vi "bulk_read.vi"() -> ()   [LabVIEW 2016]
uses:
  dxl_x86_c.lvlib/dxl_x86_c.lvlib
panel:
  out "dynamixel_comm_result":string
  out "dynamixel_error":string
  in  "LEN_MX_\nMOVING":u16=1
  in  "ADDR_MX_\nMOVING":u16=46
  out "value : MX (LED)\nis moving 2":bool
  out "group_num":i32
  in  "LEN_MX_\nPRESENT_POSITION":u16=2
  in  "dynamixe2_id":u8=2
  in  "device_name":string="COM1"
  in  "ADDR_MX_\nPRESENT_POSITION":u16=36
  in  "ADDR_MX_\nGOAL_POSITION":u16=30
  in  "ADDR_MX_\nTORQUE_ENABLE":u16=24
  out "protocol_version":dbl=1.0
  out "value : MX (knob)\npresent position 1":u32(knob)
  in  "terminate":bool
  out "port_num":i32
  in  "value : MX (dial)\ngoal position":u16(knob)
  in  "dynamixel1_id":u8=1
  in  "baud_rate":i32=57600
  # "/*******************************************************************************\n* Copyright (c) 2016, ROBOTIS CO., LTD.\n* All rights reserved.\n*\n* Redistribution and use in source and binary forms, with or without\n* modification, are permitted provided that the following conditions are met:\n*\n* * Redistributions of source code must retain the above copyright notice, this\n*   list of conditions and the following disclaimer.\n*\n* * Redistributions in binary form must reproduce the above copyright notice,\n*   this list of conditions and the following disclaimer in the documentation\n*   and/or other materials provided with the distribution.\n*\n* * Neither the name of ROBOTIS nor the names of its\n*   contributors may be used to endorse or promote products derived from\n*   this software without specific prior written permission.\n*\n* THIS SOFTWARE IS PROVIDED BY THE COPYRIGHT HOLDERS AND CONTRIBUTORS \"AS IS\"\n* AND ANY EXPRESS OR IMPLIED WARRANTIES, INCLUDING, BUT NOT LIMITED TO, THE\n* IMPLIED WARRANTIES OF MERCHANTABILITY AND FITNESS FOR A PARTICULAR PURPOSE ARE\n* DISCLAIMED. IN NO EVENT SHALL THE COPYRIGHT HOLDER OR CONTRIBUTORS BE LIABLE\n* FOR ANY DIRECT, INDIRECT, INCIDENTAL, SPECIAL, EXEMPLARY, OR CONSEQUENTIAL\n* DAMAGES (INCLUDING, BUT NOT LIMITED TO, PROCUREMENT OF SUBSTITUTE GOODS OR\n* SERVICES; LOSS OF USE, DATA, OR PROFITS; OR BUSINESS INTERRUPTION) HOWEVER\n* CAUSED AND ON ANY THEORY OF LIABILITY, WHETHER IN CONTRACT, STRICT LIABILITY,\n* OR TORT (INCLUDING NEGLIGENCE OR OTHERWISE) ARISING IN ANY WAY OUT OF THE USE\n* OF THIS SOFTWARE, EVEN IF ADVISED OF THE POSSIBILITY OF SUCH DAMAGE.\n*******************************************************************************/\n\n/* Author: Ryu Woon Jung (Leon) */"
  # "Available Dynamixel model on this example : All models using Protocol 1.0\nThis example is designed for using two Dynamixel MX-28s, and an USB2DYNAMIXEL.\nTo use another Dynamixel model, such as X series, see their details in E-Manual(support.robotis.com) \n   and edit \"numeric control\"s seen left with \"Edit Text\" tool.\nBe sure that Dynamixel MX properties are already set as %% ID : 1 / Baudnum : 34 (Baudrate : 57600)\n\n1. Run example by click above \"Run\" button (below \"Edit\" menu).\n2. Drag \"dial\" then you may see the Dynamixel and \"knob\"s rotating\n3. To finish the example, press \"terminate\" button."
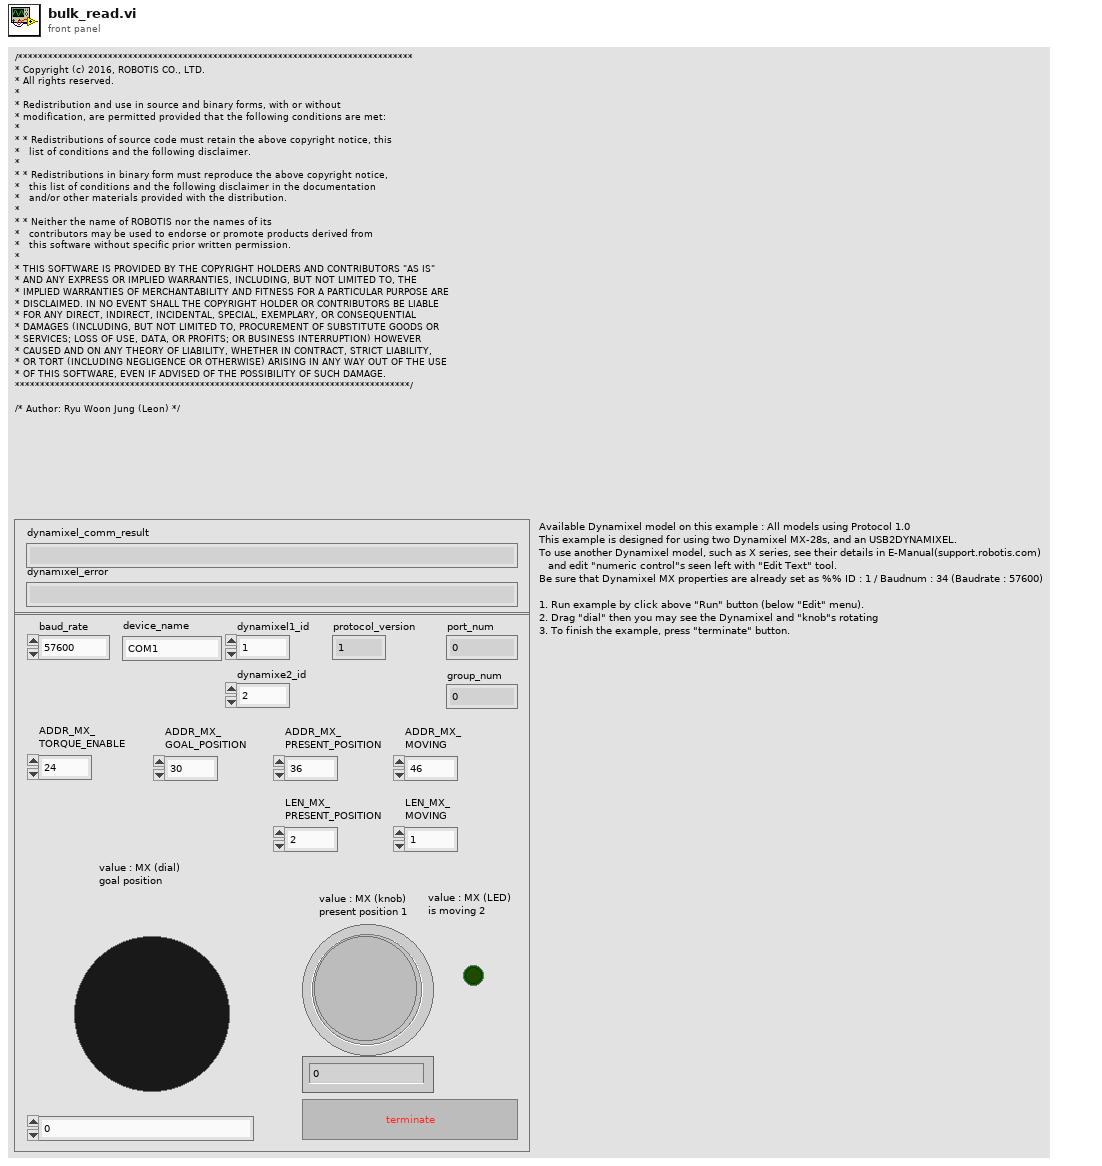
[diagram p1: front panel]
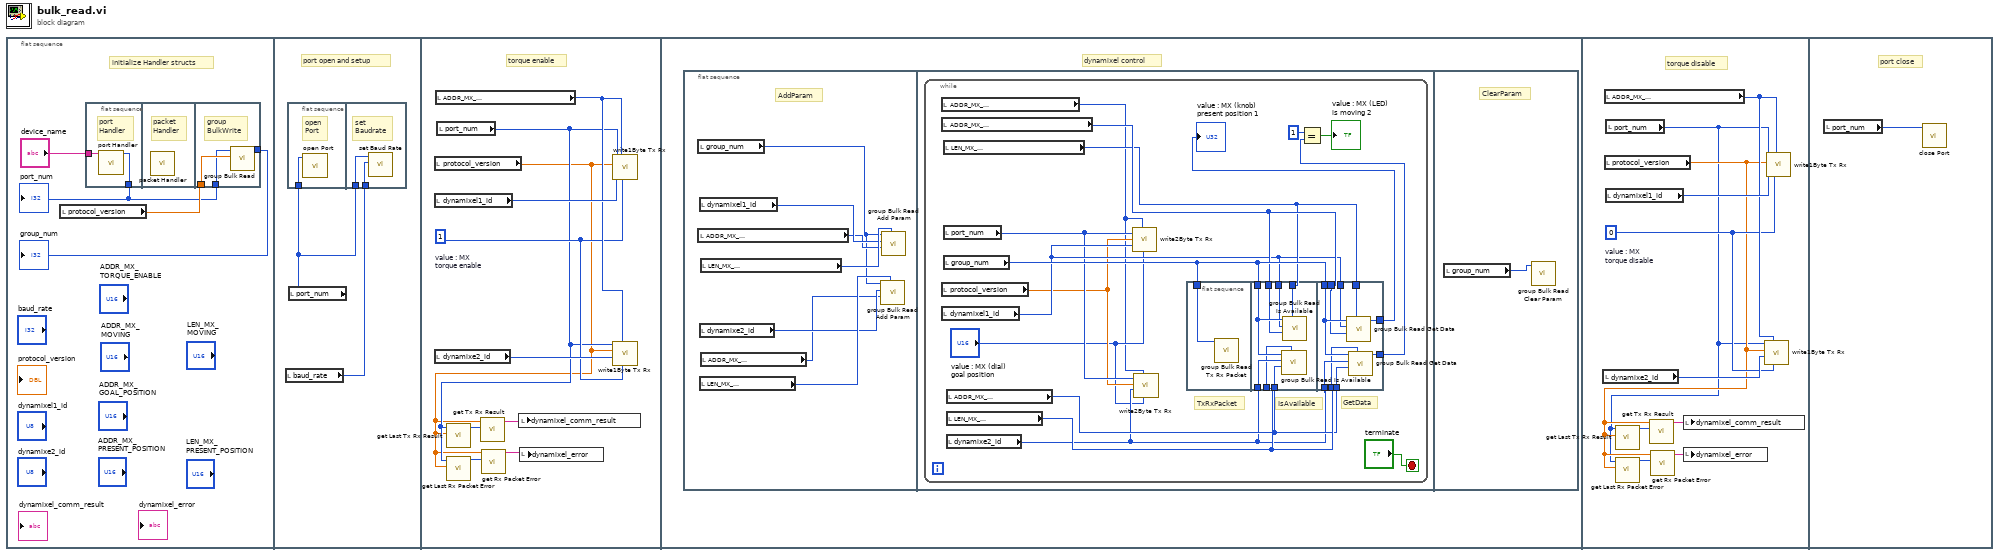
[diagram p0: block diagram]
diagram:
  n1 = flat-sequence {
    frame #0 {
      # "initialize Handler structs"
      n2 = local read "protocol_version"() -> (w3:dbl)
      n3 = flat-sequence {
        tunnel: "device_name" -> [w6]
        tunnel: [w5] -> w2
        tunnel: w3 -> [w9]
        tunnel: w2 -> [w8]
        tunnel: [w7] -> w1
        frame #0 {
          # "port\nHandler"
          n4 = call "port Handler.vi"("port_name"=w6) -> ("function return"=w5:i32)  [unwired: 10 in]
        }
        frame #1 {
          # "packet\nHandler"
          n5 = call "packet Handler.vi"() -> ()  [unwired: 12 in]
        }
        frame #2 {
          # "group\nBulkWrite"
          n6 = call "group Bulk Read.vi"("protocol_version"=w9, "port_num"=w8) -> ("function return"=w7:i32)  [unwired: 9 in]
        }
      }
      "port_num" <- w2
      "group_num" <- w1
    }
    frame #1 {
      # "port open and setup"
      n7 = local read "baud_rate"() -> (w10:i32)
      n8 = flat-sequence {
        tunnel: w11 -> [w12]
        tunnel: w11 -> [w14]
        tunnel: w10 -> [w13]
        frame #0 {
          # "open\nPort"
          n9 = call "open Port.vi"("port_num"=w12) -> ()  [unwired: 10 in, 1 out]
        }
        frame #1 {
          # "set\nBaudrate"
          n10 = call "set Baud Rate.vi"("baudrate"=w13, "port_num"=w14) -> ()  [unwired: 9 in, 1 out]
        }
      }
      n11 = local read "port_num"() -> (w11:i32)
    }
    frame #2 {
      w21 = 1  # value : MX torque enable
      # "torque enable"
      n12 = local read "protocol_version"() -> (w15:dbl)
      n13 = local read "dynamixel1_id"() -> (w24:u8)
      n14 = local read "dynamixe2_id"() -> (w22:u8)
      n15 = local read "ADDR_MX_\nTORQUE_ENABLE"() -> (w23:u16)
      n16 = local read "port_num"() -> (w16:i32)
      n17 = call "get Last Tx Rx Result.vi"("protocol_version"=w15, "port_num"=w16) -> ("function return"=w17:i32)  [unwired: 9 in]
      n18 = call "get Last Rx Packet Error.vi"("protocol_version"=w15, "port_num"=w16) -> ("function return"=w18:u8)  [unwired: 9 in]
      n19 = call "get Tx Rx Result.vi"("result"=w17, "protocol_version"=w15) -> ("function return"=w19:string)  [unwired: 9 in]
      n20 = call "get Rx Packet Error.vi"("error"=w18, "protocol_version"=w15) -> ("function return"=w20:string)  [unwired: 9 in]
      n21 = local write "dynamixel_comm_result"(w19) -> ()
      n22 = local write "dynamixel_error"(w20) -> ()
      n23 = call "write1Byte Tx Rx.vi"("data"=w21, "address"=w23, "id"=w24, "protocol_version"=w15, "port_num"=w16) -> ()  [unwired: 7 in]
      n24 = call "write1Byte Tx Rx.vi"("data"=w21, "address"=w23, "id"=w22, "protocol_version"=w15, "port_num"=w16) -> ()  [unwired: 7 in]
    }
    frame #3 {
      # "dynamixel control"
      n25 = flat-sequence {
        frame #0 {
          # "AddParam"
          n26 = local read "group_num"() -> (w27:i32)
          n27 = local read "ADDR_MX_\nPRESENT_POSITION"() -> (w29:u16)
          n28 = local read "dynamixel1_id"() -> (w30:u8)
          n29 = local read "dynamixe2_id"() -> (w26:u8)
          n30 = local read "LEN_MX_\nMOVING"() -> (w28:u16)
          n31 = local read "LEN_MX_\nPRESENT_POSITION"() -> (w31:u16)
          n32 = local read "ADDR_MX_\nMOVING"() -> (w25:u16)
          n33 = call "group Bulk Read Add Param.vi"("data_length"=w28, "start_address"=w25, "id"=w26, "group_num"=w27) -> ()  [unwired: 7 in, 1 out]
          n34 = call "group Bulk Read Add Param.vi"("data_length"=w31, "start_address"=w29, "id"=w30, "group_num"=w27) -> ()  [unwired: 7 in, 1 out]
        }
        frame #1 {
          n35 = while {
            stop <- "terminate" stop-if-true
            # "TxRxPacket"
            # "IsAvailable"
            # "GetData"
            n36 = local read "ADDR_MX_\nGOAL_POSITION"() -> (w32:u16)
            n37 = local read "ADDR_MX_\nPRESENT_POSITION"() -> (w45:u16)
            n38 = local read "protocol_version"() -> (w35:dbl)
            n39 = local read "dynamixel1_id"() -> (w37:u8)
            n40 = local read "LEN_MX_\nPRESENT_POSITION"() -> (w38:u16)
            n41 = local read "port_num"() -> (w36:i32)
            n42 = local read "group_num"() -> (w46:i32)
            n43 = local read "ADDR_MX_\nMOVING"() -> (w39:u16)
            n44 = local read "LEN_MX_\nMOVING"() -> (w44:u16)
            n45 = local read "dynamixe2_id"() -> (w34:u8)
            n46 = call "write2Byte Tx Rx.vi"("data"="value : MX (dial)\ngoal position", "address"=w32, "id"=w37, "protocol_version"=w35, "port_num"=w36) -> ()  [unwired: 7 in]
            n47 = call "write2Byte Tx Rx.vi"("data"="value : MX (dial)\ngoal position", "address"=w32, "id"=w34, "protocol_version"=w35, "port_num"=w36) -> ()  [unwired: 7 in]
            n48 = flat-sequence {
              tunnel: w46 -> [w48]
              tunnel: w46 -> [w55]
              tunnel: w34 -> [w54]
              tunnel: w45 -> [w53]
              tunnel: w44 -> [w52]
              tunnel: w39 -> [w51]
              tunnel: w38 -> [w50]
              tunnel: w37 -> [w49]
              tunnel: w46 -> [w64]
              tunnel: w34 -> [w63]
              tunnel: w45 -> [w62]
              tunnel: w44 -> [w59]
              tunnel: [w61] -> w41
              tunnel: [w60] -> w40
              tunnel: w39 -> [w58]
              tunnel: w38 -> [w57]
              tunnel: w37 -> [w56]
              frame #0 {
                n49 = call "group Bulk Read Tx Rx Packet.vi"("group_num"=w48) -> ()  [unwired: 11 in]
              }
              frame #1 {
                n50 = call "group Bulk Read Is Available.vi"("data_length"=w52, "address"=w51, "id"=w54, "group_num"=w55) -> ()  [unwired: 7 in, 1 out]
                n51 = call "group Bulk Read Is Available.vi"("data_length"=w50, "address"=w53, "id"=w49, "group_num"=w55) -> ()  [unwired: 7 in, 1 out]
              }
              frame #2 {
                n52 = call "group Bulk Read Get Data.vi"("data_length"=w57, "address"=w62, "id"=w56, "group_num"=w64) -> ("function return"=w60:u32)  [unwired: 7 in]
                n53 = call "group Bulk Read Get Data.vi"("data_length"=w59, "address"=w58, "id"=w63, "group_num"=w64) -> ("function return"=w61:u32)  [unwired: 7 in]
              }
            }
            n54 = Equal?(x=1, y=w41) -> (x = y?=→"value : MX (LED)\nis moving 2":bool)
            "value : MX (knob)\npresent position 1" <- w40
          }
        }
        frame #2 {
          # "ClearParam"
          n55 = local read "group_num"() -> (w65:i32)
          n56 = call "group Bulk Read Clear Param.vi"("group_num"=w65) -> ()  [unwired: 11 in]
        }
      }
    }
    frame #4 {
      w72 = 0  # value : MX torque disable
      # "torque disable"
      n57 = local read "dynamixe2_id"() -> (w73:u8)
      n58 = local read "ADDR_MX_\nTORQUE_ENABLE"() -> (w74:u16)
      n59 = local read "protocol_version"() -> (w67:dbl)
      n60 = local read "dynamixel1_id"() -> (w75:u8)
      n61 = local read "port_num"() -> (w66:i32)
      n62 = call "get Last Tx Rx Result.vi"("protocol_version"=w67, "port_num"=w66) -> ("function return"=w69:i32)  [unwired: 9 in]
      n63 = call "get Last Rx Packet Error.vi"("protocol_version"=w67, "port_num"=w66) -> ("function return"=w68:u8)  [unwired: 9 in]
      n64 = call "get Tx Rx Result.vi"("result"=w69, "protocol_version"=w67) -> ("function return"=w70:string)  [unwired: 9 in]
      n65 = call "get Rx Packet Error.vi"("error"=w68, "protocol_version"=w67) -> ("function return"=w71:string)  [unwired: 9 in]
      n66 = local write "dynamixel_comm_result"(w70) -> ()
      n67 = local write "dynamixel_error"(w71) -> ()
      n68 = call "write1Byte Tx Rx.vi"("data"=w72, "address"=w74, "id"=w73, "protocol_version"=w67, "port_num"=w66) -> ()  [unwired: 7 in]
      n69 = call "write1Byte Tx Rx.vi"("data"=w72, "address"=w74, "id"=w75, "protocol_version"=w67, "port_num"=w66) -> ()  [unwired: 7 in]
    }
    frame #5 {
      # "port close"
      n70 = local read "port_num"() -> (w76:i32)
      n71 = call "close Port.vi"("port_num"=w76) -> ()  [unwired: 11 in]
    }
  }
